vi "Config Spark Max Output HW Get Set.vi"(6 "Get(f) Set(t)":bool, 7 "SparkMax Output":T1, 8 "Error":errorcluster, 11 "Drive Refs":T2) -> (0 "Error Out":errorcluster, 3 "Drive Refs Out":T2, 5 "SparkMax Output Out":T1)   [LabVIEW 2020, in "Swerve AM_ACT.lvlib"]
uses:
  Swerve AM_ACT.lvlib
  <vilib>/Rock Robotics/WPI/MotorControl/WPI_MotorControlDeviceRef.ctl
  <vilib>/Rock Robotics/WPI/MotorControl/WPI_MotorControlType.ctl
  <vilib>/Rock Robotics/SystemInterfaces/DIO/FPGA_DIOPWMChannel.ctl
  <vilib>/Rock Robotics/WPI/PWM/WPI_PWMDeadband.ctl
  <vilib>/Rock Robotics/SystemInterfaces/DIO/FPGA_DIOChannel.ctl
  Shared Code/TypeDefs/Cluster_Config Spark Max Motor Output.ctl
  <vilib>/Utility/Data Type/NI_Data Type.lvlib
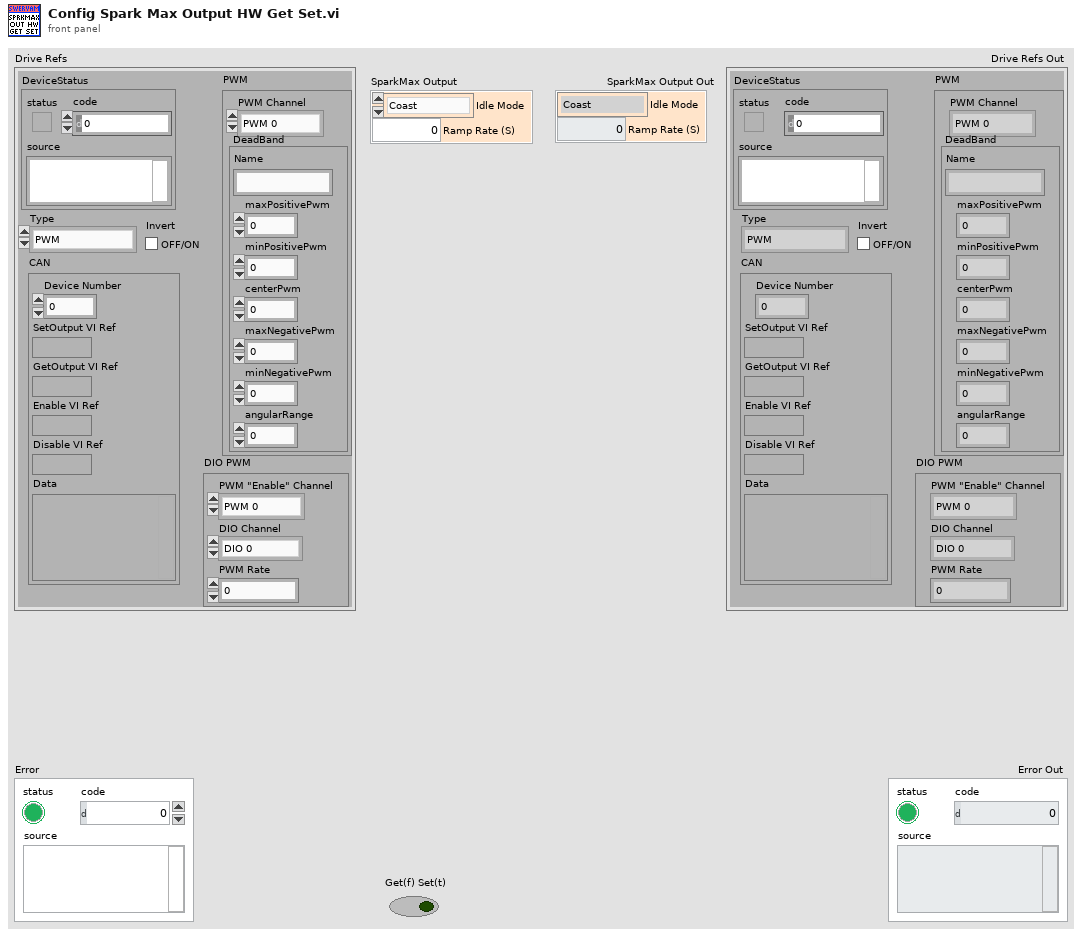
[diagram p1: front panel]
types:
  T1 = typedef "Cluster_Config Spark Max Motor Output.ctl" = cluster{"Idle Mode":enum16{"Coast", "Brake"}, "Ramp Rate (S)":dbl}
  T2 = typedef "WPI_MotorControlDeviceRef.ctl" = cluster{"DeviceStatus":errorcluster, "Type":T3, "PWM":cluster{"PWM Channel":T4, "DeadBand":T5}, "CAN":cluster{"Device Number":u8, "SetOutput VI Ref":variant, "GetOutput VI Ref":variant, "Enable VI Ref":variant, "Disable VI Ref":variant, "Data":variant}, "Invert":bool, "DIO PWM":cluster{"PWM \"Enable\" Channel":T4, "DIOChannel":T6, "PWM Rate":dbl}}
  T3 = typedef "WPI_MotorControlType.ctl" = enum16{"PWM", "CAN", "DIO PWM"}
  T4 = typedef "FPGA_DIOPWMChannel.ctl" = enum8{"PWM 0", "PWM 1", "PWM 2", "PWM 3", "PWM 4", "PWM 5", "PWM 6", "PWM 7", "PWM 8", "PWM 9", "PWM MXP 0", "PWM MXP 1", "PWM MXP 2", "PWM MXP 3", "PWM MXP 4", "PWM MXP 5", "PWM MXP 6", "PWM MXP 7", "PWM MXP 8", "PWM MXP 9", "Invalid"}
  T5 = typedef "WPI_PWMDeadband.ctl" = cluster{"Name":string, "maxPositivePwm":i32, "minPositivePwm":i32, "centerPwm":i32, "maxNegativePwm":i32, "minNegativePwm":i32, "angularRange":u16}
  T6 = typedef "FPGA_DIOChannel.ctl" = enum8{"DIO 0", "DIO 1", "DIO 2", "DIO 3", "DIO 4", "DIO 5", "DIO 6", "DIO 7", "DIO 8", "DIO 9", "DIO MXP 0", "DIO MXP 1", "DIO MXP 2", "DIO MXP 3", "DIO MXP 4", "DIO MXP 5", "DIO MXP 6", "DIO MXP 7", "DIO MXP 8", "DIO MXP 9", "DIO MXP 10", "DIO MXP 11", "DIO MXP 12", "DIO MXP 13", "DIO MXP 14", "DIO MXP 15", "SPI Port CS1", "SPI Port CS2", "SPI Port CS3", "SPI Port MISO", "SPI Port MOSI", "Invalid"}
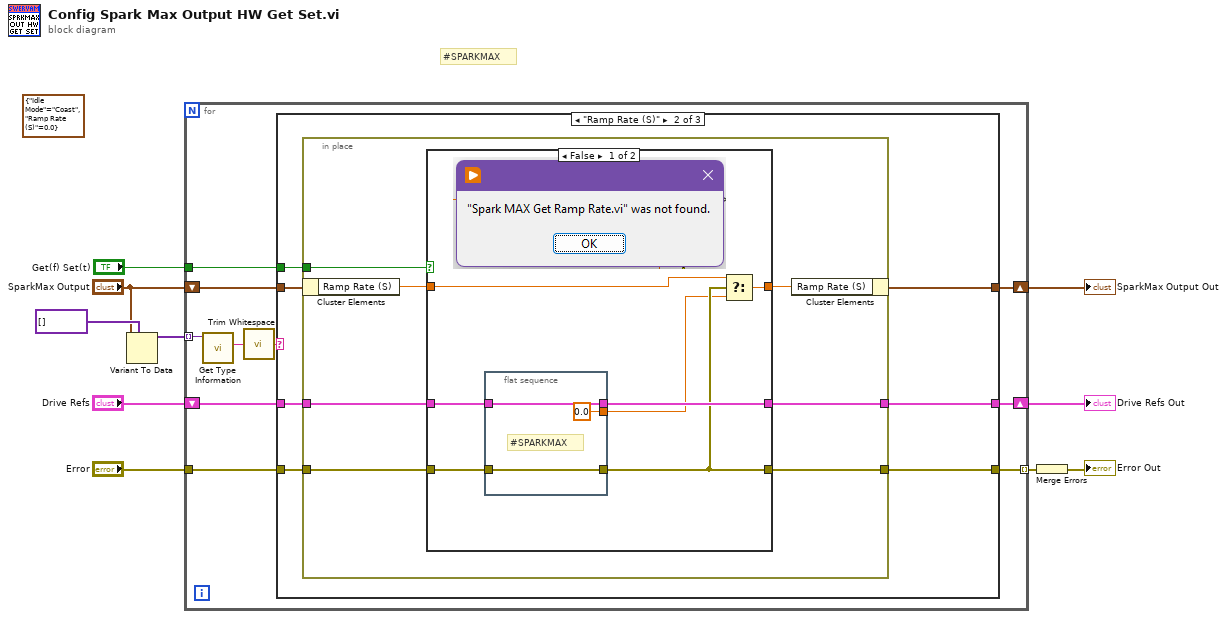
[diagram p0: block diagram]
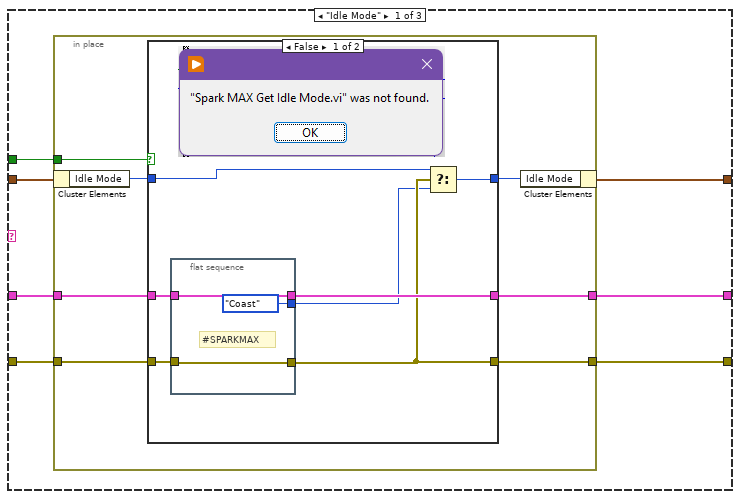
[diagram p2: hidden frame]
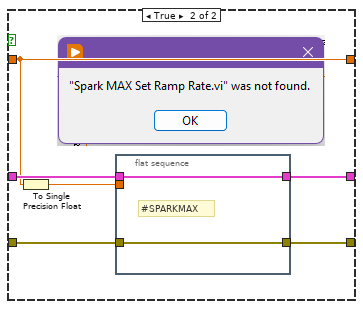
[diagram p4: hidden frame]
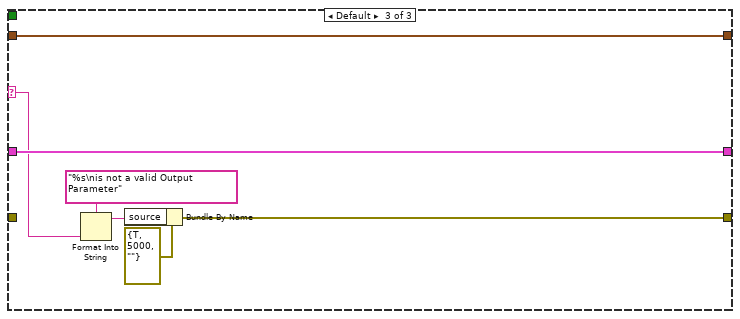
[diagram p5: hidden frame]
diagram:
  (unwired) T1 {"Idle Mode"=enum."Coast", "Ramp Rate (S)"=0.0} ("SparkMax Output")
  # "#SPARKMAX"
  n1 = Variant To Data(type=variant[] [], Variant="SparkMax Output") -> (data=w5:variant[])  [unwired: 1 in, 1 out]
  n2 = for {
    shift-right: [w11] -> w10
    shift-left: "SparkMax Output" -> [w17]
    shift-right: [w12] -> w8
    shift-left: "Drive Refs" -> [w16]
    tunnel: "Get(f) Set(t)" -> [w15]
    tunnel: w5 -> [w19] mode=indexing
    tunnel: "Error" -> [w14]
    tunnel: [w13] -> w2 mode=indexing
    n3 = call <vilib>:"Get Type Information.vi"("variant"=w19) -> ("name"=w20:string)  [unwired: 6 in, 4 out]
    n4 = call <vilib>:"Trim Whitespace.vi"("string"=w20) -> ("trimmed string"=w18:string)  [unwired: 1 in]
    n5 = case shown="\"Ramp Rate (S)\"" w18 {
      selector: w18 -> [_ _ w88]
      tunnel: w17 -> [w27 w58 w90]
      tunnel: w16 -> [w23 w54 w89]
      tunnel: w15 -> [w26 w57 _]
      tunnel: w14 -> [w25 w56 _]
      tunnel: [w24 w55 w86] -> w13
      tunnel: [w22 w53 w89] -> w12
      tunnel: [w21 w52 w90] -> w11
      frame "Idle Mode" {
        n6 = in-place {
          in-place-border: w26 -> [w34]
          in-place-border: w25 -> [w32]
          in-place-border: [w31] -> w24
          in-place-border: w23 -> [w30]
          in-place-border: [w29] -> w22
          n7 = in-place-cluster #1(w27) -> ("Idle Mode"=w33:enum16{"Coast", "Brake"})
          n8 = case shown="False" w34 {
            tunnel: w33 -> [w37 w47]
            tunnel: w32 -> [w39 w45]
            tunnel: [w38 w46] -> w31
            tunnel: w30 -> [w41 w49]
            tunnel: [w40 w48] -> w29
            tunnel: [w35 w47] -> w28
            frame False {
              n9 = flat-sequence {
                tunnel: w41 -> [w44]
                tunnel: [w44] -> w40
                tunnel: w39 -> [w42]
                tunnel: [w42] -> w38
                tunnel: [enum16{"Coast", "Brake"}."Coast" ("Idle Mode")] -> w36
                frame #0 {
                  # "#SPARKMAX"
                }
              }
              n10 = Select(t=w37, s=w38, f=w36) -> (s? t:f=w35:enum16{"Coast", "Brake"})
            }
            frame True {
              n11 = flat-sequence {
                tunnel: w49 -> [w50]
                tunnel: [w50] -> w48
                tunnel: w47 -> [_]
                tunnel: [w51] -> w46
                tunnel: w45 -> [w51]
                frame #0 {
                  # "#SPARKMAX"
                }
              }
            }
          }
          n12 = in-place-cluster #1("Idle Mode"=w28) -> (w21:T1)
        }
      }
      frame "Ramp Rate (S)" {
        n13 = in-place {
          in-place-border: w57 -> [w65]
          in-place-border: w56 -> [w63]
          in-place-border: [w62] -> w55
          in-place-border: w54 -> [w61]
          in-place-border: [w60] -> w53
          n14 = in-place-cluster #2(w58) -> ("Ramp Rate (S)"=w64:dbl)
          n15 = case shown="False" w65 {
            tunnel: w64 -> [w68 w79]
            tunnel: w63 -> [w70 w77]
            tunnel: [w69 w78] -> w62
            tunnel: w61 -> [w72 w81]
            tunnel: [w71 w80] -> w60
            tunnel: [w66 w79] -> w59
            frame False {
              n16 = flat-sequence {
                tunnel: w72 -> [w75]
                tunnel: [w75] -> w71
                tunnel: w70 -> [w74]
                tunnel: [w74] -> w69
                tunnel: [0.0 ("Ramp Rate")] -> w67
                frame #0 {
                  # "#SPARKMAX"
                }
              }
              n17 = Select(t=w68, s=w69, f=w67) -> (s? t:f=w66:dbl)
            }
            frame True {
              n18 = To Single Precision Float(number=w79) -> (single precision float=w76:sgl)
              n19 = flat-sequence {
                tunnel: w81 -> [w82]
                tunnel: [w82] -> w80
                tunnel: [w83] -> w78
                tunnel: w77 -> [w83]
                tunnel: w76 -> [_]
                frame #0 {
                  # "#SPARKMAX"
                }
              }
            }
          }
          n20 = in-place-cluster #2("Ramp Rate (S)"=w59) -> (w52:T1)
        }
      }
      frame Default {
        n21 = Format Into String(format string="%s\nis not a valid Output Parameter", w88) -> (resulting string=w84:string)  [unwired: 2 in, 1 out]
        n22 = Bundle By Name(cluster=errorcluster {"status"=TRUE, "code"=5000, "source"=""} ("error out"), "source"=w84) -> (w86:errorcluster)
      }
    }
  }
  "Drive Refs Out" <- w8
  "SparkMax Output Out" <- w10
  n23 = Merge Errors(w2) -> (→"Error Out":errorcluster)
